vi "Time string to time stamp.vi"(8 "error in (no error)":errorcluster, 10 "Time String":string, 11 "OLE DB Timestamp in":refnum<class "OLE DB Timestamp.lvclass">) -> (0 "error out":errorcluster, 2 "Time Stamp":timestamp, 3 "OLE DB Timestamp out":refnum<class "OLE DB Timestamp.lvclass">)   [LabVIEW 2020, in "Basic Columns.lvlib" / "OLE DB Timestamp.lvclass"]
uses:
  OLE DB Timestamp.lvclass
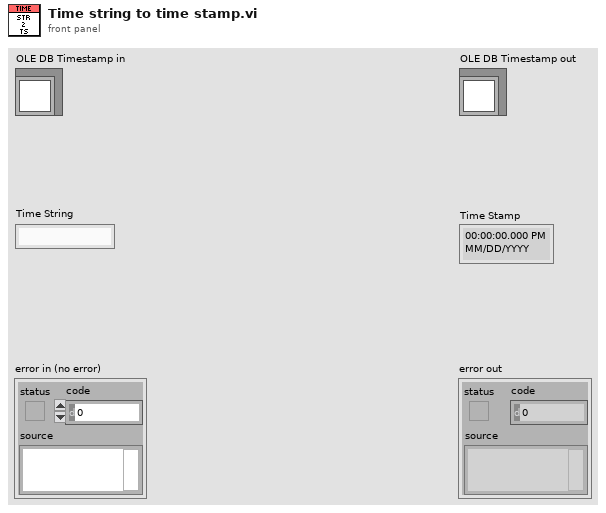
[diagram p1: front panel]
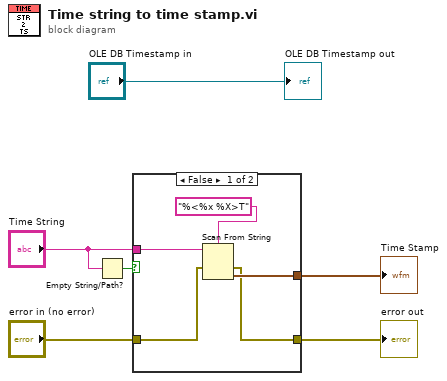
[diagram p0: block diagram]
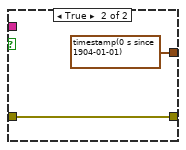
[diagram p2: hidden frame]
diagram:
  n1 = Empty String/Path?(string/path="Time String") -> (empty?=w2:bool)
  n2 = case shown="False" w2 {
    tunnel: "Time String" -> [w10 _]
    tunnel: [w9 timestamp(0 s since 1904-01-01)] -> w5
    tunnel: "error in (no error)" -> [w8 w12]
    tunnel: [w7 w12] -> w3
    frame False {
      n3 = Scan From String(format string="%<%x %X>T", input string=w10, error in=w8) -> (error out=w7:errorcluster, output 1=w9:timestamp)  [unwired: 2 in, 2 out]
    }
    frame True {
    }
  }
  "error out" <- w3
  "Time Stamp" <- w5
  "OLE DB Timestamp out" <- "OLE DB Timestamp in"
